vi "Write Open plot.vi"(8 "error in (no error)":errorcluster, 10 "Open plot":bool, 11 "Pulse Acquired Result in":refnum<class "Pulse Acquired Result.lvclass">) -> (0 "error out":errorcluster, 3 "Pulse Acquired Result out":refnum<class "Pulse Acquired Result.lvclass">)   [LabVIEW 2016, in "Pulse Acquired Result.lvclass"]
uses:
  Pulse Acquired Result.lvclass
  Pulse Acquired Result.lvclass/Pulse Acquired Result.ctl
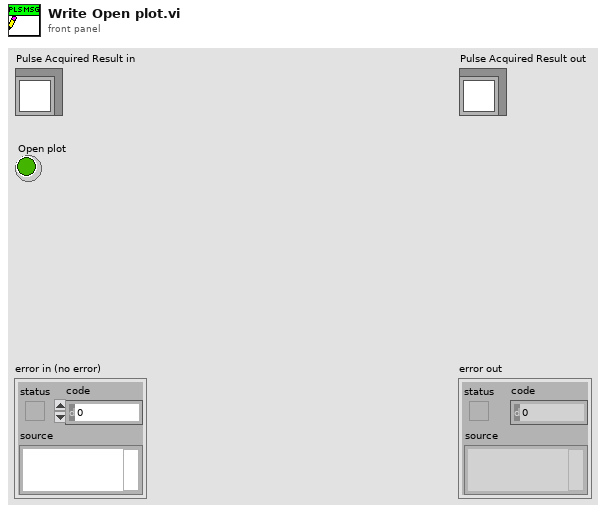
[diagram p1: front panel]
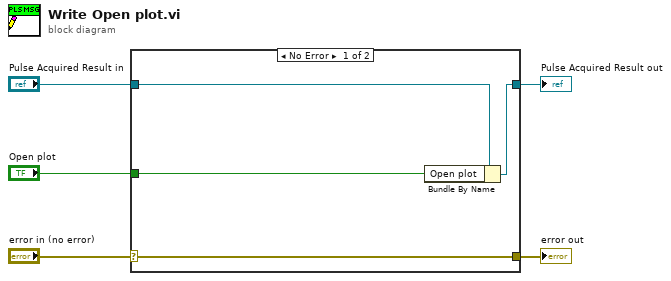
[diagram p0: block diagram]
diagram:
  n1 = case shown="No Error" "error in (no error)" {
    selector: "error in (no error)" -> [w9 w10]
    tunnel: [w9 w10] -> w4
    tunnel: [w7 w11] -> w2
    tunnel: "Pulse Acquired Result in" -> [w8 w11]
    tunnel: "Open plot" -> [w6 _]
    frame No Error {
      n2 = Bundle By Name(cluster=w8, "Open plot"=w6) -> (w7:refnum<class "Pulse Acquired Result.lvclass">)
    }
    frame Error {
    }
  }
  "error out" <- w4
  "Pulse Acquired Result out" <- w2
